vi "Periodic Tasks (Conley Anderson's conflicted copy 2015-02-02).vi"(8 "error in":errorcluster) -> ()   [LabVIEW 2013]
doc: "This VI runs in parallel to other tasks. It can contain as many user-defined periodic loops as you need. These can carry out PID or other sorts of timed response."
uses:
  <vilib>/Rock Robotics/WPI/DriverStation/WPI_DriverStationRobotMode2.ctl
  <vilib>/Rock Robotics/SystemInterfaces/Utilities/FPGA_UtilitiesLED Source.ctl
  <vilib>/Rock Robotics/SystemInterfaces/Utilities/FPGA_UtilitiesLED State.ctl
  <vilib>/Rock Robotics/WPI/Solenoid/WPI_SolenoidValue.ctl
  <vilib>/Rock Robotics/WPI/Relay/WPI_RelayValue.ctl
  <vilib>/Rock Robotics/WPI/Compressor/WPI_CompressorGetSetRefNum.vi
  Robot Global Data.vi
  <vilib>/Rock Robotics/WPI/Joystick/WPI_JoystickGetSetRefNum.vi
  <vilib>/Rock Robotics/WPI/Solenoid/WPI_SolenoidSetEnum.vi
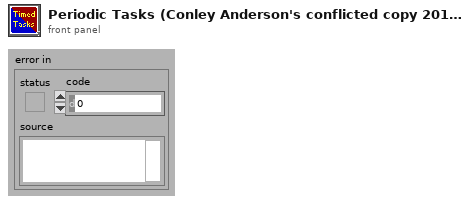
[diagram p1: front panel]
types:
  T1 = typedef "FPGA_UtilitiesLED State.ctl" = enum16{"Off", "On", "Toggle"}
  T2 = typedef "FPGA_UtilitiesLED Source.ctl" = enum16{"User LED", "FPGA LED"}
  T3 = typedef "WPI_AnalogChannelDevRef.ctl" = cluster{"DevStatus":errorcluster, "Analog Module":T4, "Analog Channel":T5}
  T4 = typedef "FPGA_TypedefAnalogModule.ctl" = enum16{"Analog Module 1", "Analog Module 2"}
  T5 = typedef "FPGA_AIChannel.ctl" = enum8{"AI 1", "AI 2", "AI 3", "AI 4", "AI 5", "AI 6", "AI 7", "AI 8", "Invalid"}
  T6 = typedef "WPI_RelayDevRef.ctl" = cluster{"DevStatus":errorcluster, "Relay Channel":T7, "Digital Module":T8, "Relay Direction":T9}
  T7 = typedef "FPGA_DIORelayChannel.ctl" = enum8{"Relay 1", "Relay 2", "Relay 3", "Relay 4", "Relay 5", "Relay 6", "Relay 7", "Relay 8", "Invalid"}
  T8 = typedef "FPGA_TypedefDigitalModule.ctl" = enum16{"Digital Module 1", "Digital Module 2"}
  T9 = typedef "WPI_RelayDirection.ctl" = enum16{"Both directions", "Forward only", "Reverse only"}
  T10 = typedef "WPI_DigitalInputDevRef.ctl" = cluster{"DevStatus":errorcluster, "DIO Channel":T11, "Digital Module":T8}
  T11 = typedef "FPGA_DIOChannel.ctl" = enum8{"DIO 1", "DIO 2", "DIO 3", "DIO 4", "DIO 5", "DIO 6", "DIO 7", "DIO 8", "DIO 9", "DIO 10", "DIO 11", "DIO 12", "DIO 13", "DIO 14", "Invalid"}
  T12 = typedef "WPI_SolenoidDevRef.ctl" = cluster{"DevStatus":errorcluster, "Solenoid Module":T13, "Forward Solenoid Channel":T14, "Reverse Solenoid Channel":T14}
  T13 = typedef "FPGA_TypedefSolenoidModule.ctl" = enum16{"Solenoid Module 1", "Solenoid Module 2"}
  T14 = typedef "WPI_SolenoidChannel.ctl" = enum8{"Solenoid 1", "Solenoid 2", "Solenoid 3", "Solenoid 4", "Solenoid 5", "Solenoid 6", "Solenoid 7", "Solenoid 8", "Invalid"}
  T15 = typedef "WPI_JoystickDevRef.ctl" = cluster{"Device":T16}
  T16 = typedef "WPI_JoystickDeviceEnum.ctl" = enum16{"USB 1", "USB 2", "USB 3", "USB 4", "Kinect 1", "Kinect 2"}
  T17 = typedef "WPI_MotorControlDeviceRef.ctl" = cluster{"DeviceStatus":errorcluster, "Type":enum16{"PWM", "CAN"}, "PWM":cluster{"Digital Module":T8, "PWM Channel":T18, "DeadBand":T19}, "CAN":cluster{"Device Number":u8, "Control Mode":T20, "Semaphore":T21, "Max Vout":dbl}, "Invert":bool, "TransformRef":T22, "InvTransformRef":T22}
  T18 = typedef "FPGA_DIOPWMChannel.ctl" = enum8{"PWM 1", "PWM 2", "PWM 3", "PWM 4", "PWM 5", "PWM 6", "PWM 7", "PWM 8", "PWM 9", "PWM 10", "Invalid"}
  T19 = typedef "WPI_PWMDeadband.ctl" = cluster{"Name":string, "maxPositivePwm":i32, "minPositivePwm":i32, "centerPwm":i32, "maxNegativePwm":i32, "minNegativePwm":i32, "angularRange":u16}
  T20 = typedef "WPI_CANJaguar_ControlMode.ctl" = enum8{"Percent VBus", "Current", "Speed", "Position", "Voltage"}
  T21 = typedef "Semaphore RefNum" = refnum<k1>
  T22 = typedef "WPI_PWMTransform_ConPane.ctl" = refnum<vi>
  T23 = typedef "WPI_CompressorDevRef.ctl" = cluster{"DevStatus":errorcluster, "DigitalInputDevRef":T10, "RelayDevRef":T6}
  T24 = cluster{"JoystickDevRef":T15, "JoystickDevRef":T15, "SolenoidDevRef":T12, "SolenoidDevRef":T12, "RelayDevRef":T6, "RelayDevRef":T6, "RelayDevRef":T6, "MotorControlDevRef":T17, "MotorControlDevRef":T17, "DigitalInputDevRef":T10, "DigitalInputDevRef":T10, "AIDeviceRef":T3, "CompressorDevRef":T23}
  T25 = typedef "WPI_DriverStationRobotMode2.ctl" = enum16{"Autonomous Disabled", "Autonomous Enabled", "Teleop Disabled", "Teleop Enabled", "Timeout", "Finish", "Test Disabled", "Test Enabled"}
  T26 = typedef "WPI_RelayValue.ctl" = enum16{"Off", "On", "Forward", "Reverse"}
  T27 = typedef "WPI_SolenoidValue.ctl" = enum16{"Off", "On", "Forward", "Reverse"}
  T28 = typedef "WPI_JoystickButtonState.ctl" = cluster{"Button 1":bool, "Button 2":bool, "Button 3":bool, "Button 4":bool, "Button 5":bool, "Button 6":bool, "Button 7":bool, "Button 8":bool, "Button 9":bool, "Button 10":bool, "Button 11":bool, "Button 12":bool}
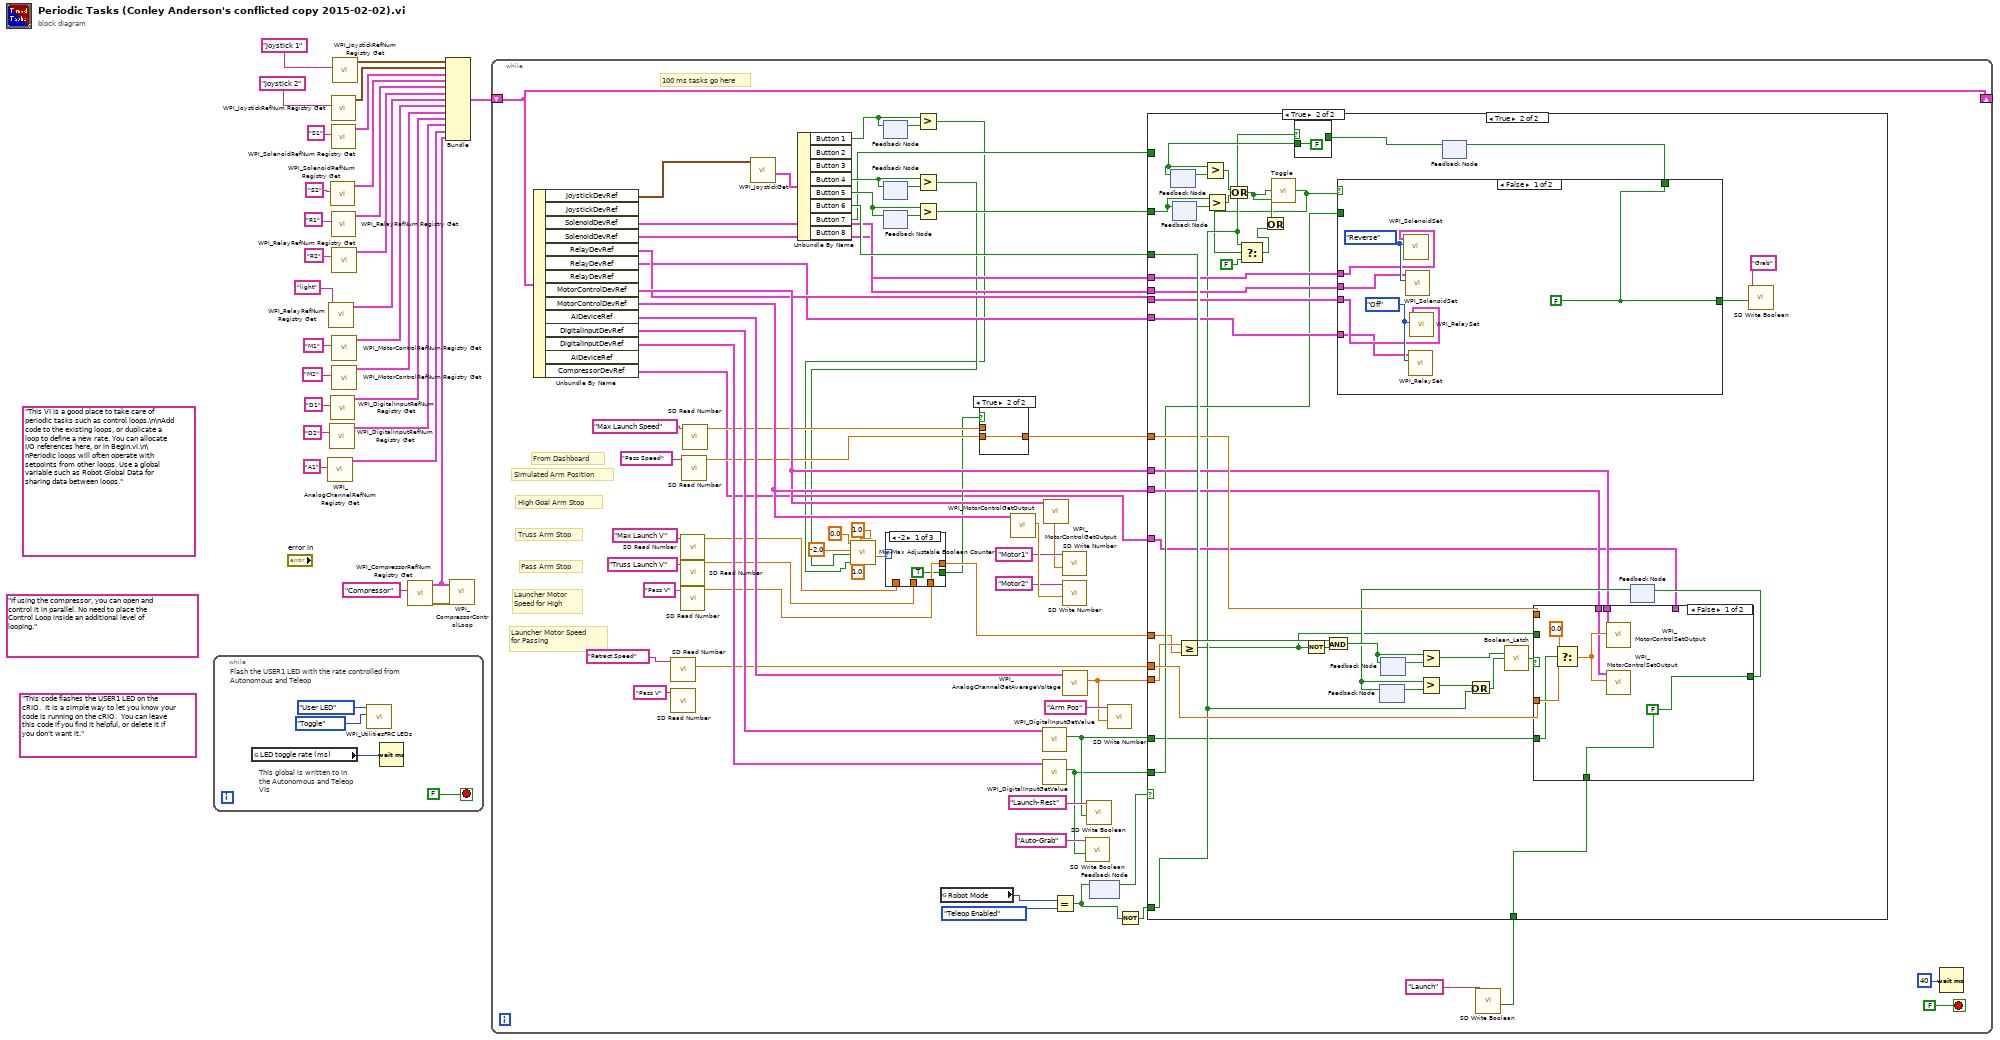
[diagram p0: block diagram]
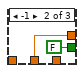
[diagram p3: hidden frame]
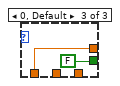
[diagram p4: hidden frame]
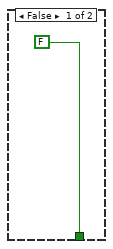
[diagram p5: hidden frame]
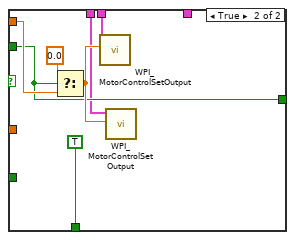
[diagram p7: hidden frame]
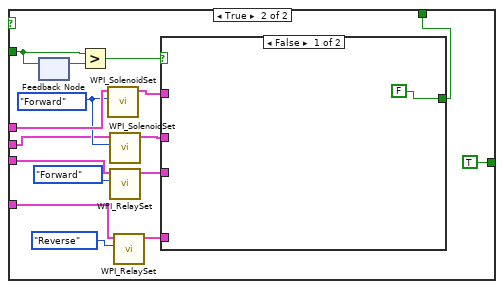
[diagram p8: hidden frame]
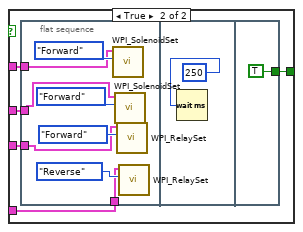
[diagram p9: hidden frame]
diagram:
  (unwired) "If using the compressor, you can open and control it in parallel. No need to place the Control Loop inside an additional level of looping."
  (unwired) "This code flashes the USER1 LED on the cRIO.  It is a simple way to let you know your code is running on the cRIO.  You can leave this code if you find it helpful, or delete it if you don't want it."
  (unwired) "This VI is a good place to take care of periodic tasks such as control loops.\n\nAdd code to the existing loops, or duplicate a loop to define a new rate. You can allocate I/O references here, or in Begin.vi.\n\nPeriodic loops will often operate with setpoints from other loops. Use a global variable such as Robot Global Data for sharing data between loops."
  n1 = while {
    stop <- FALSE stop-if-true
    # "This global is written to in the Autonomous and Teleop VIs"
    # "Flash the USER1 LED with the rate controlled from Autonomous and Teleop"
    n2 = global read "Robot Global Data.vi" "LED toggle rate (ms)"() -> (w29:u32)
    n3 = call <vilib>:"WPI_UtilitiesFRC LEDs.vi"("State"=FPGA_UtilitiesLED_State."Toggle", "LED Type"=FPGA_UtilitiesLED_Source."User LED") -> ()  [unwired: 1 in, 9 out]
    n4 = Wait (ms)(milliseconds to wait=w29) -> ()  [unwired: 1 out]
  }
  n5 = call <vilib>:"WPI_AnalogChannelRefNum Registry Get.vi"("refnum name"="A1") -> ("AIDeviceRef"=w2:T3)  [unwired: 9 in, 1 out]
  n6 = call <vilib>:"WPI_RelayRefNum Registry Get.vi"("refnum name"="light") -> ("RelayDevRef"=w10:T6)  [unwired: 9 in, 1 out]
  n7 = call <vilib>:"WPI_DigitalInputRefNum Registry Get.vi"("refnum name"="D2") -> ("DigitalInputDevRef"=w3:T10)  [unwired: 9 in, 1 out]
  n8 = call <vilib>:"WPI_SolenoidRefNum Registry Get.vi"("refnum name"="S2") -> ("SolenoidDevRef"=w13:T12)  [unwired: 9 in, 1 out]
  n9 = call <vilib>:"WPI_DigitalInputRefNum Registry Get.vi"("refnum name"="D1") -> ("DigitalInputDevRef"=w7:T10)  [unwired: 9 in, 1 out]
  n10 = call <vilib>:"WPI_JoystickRefNum Registry Get.vi"("refnum name"="Joystick 2") -> ("JoystickDevRef"=w5:T15)  [unwired: 1 in, 9 out]
  n11 = call <vilib>:"WPI_SolenoidRefNum Registry Get.vi"("refnum name"="S1") -> ("SolenoidDevRef"=w4:T12)  [unwired: 9 in, 1 out]
  n12 = call <vilib>:"WPI_RelayRefNum Registry Get.vi"("refnum name"="R1") -> ("RelayDevRef"=w12:T6)  [unwired: 9 in, 1 out]
  n13 = call <vilib>:"WPI_RelayRefNum Registry Get.vi"("refnum name"="R2") -> ("RelayDevRef"=w11:T6)  [unwired: 9 in, 1 out]
  n14 = call <vilib>:"WPI_MotorControlRefNum Registry Get.vi"("refnum name"="M1") -> ("MotorControlDevRef"=w9:T17)  [unwired: 9 in, 1 out]
  n15 = call <vilib>:"WPI_MotorControlRefNum Registry Get.vi"("refnum name"="M2") -> ("MotorControlDevRef"=w8:T17)  [unwired: 9 in, 1 out]
  n16 = call <vilib>:"WPI_JoystickRefNum Registry Get.vi"("refnum name"="Joystick 1") -> ("JoystickDevRef"=w6:T15)  [unwired: 1 in, 9 out]
  n17 = call <vilib>:"WPI_CompressorRefNum Registry Get.vi"("refnum name"="Compressor") -> ("error out"=w15:errorcluster, "CompressorDevRef"=w1:T23)  [unwired: 9 in]
  n18 = Bundle("JoystickDevRef"=w6, "JoystickDevRef"=w5, "SolenoidDevRef"=w4, "SolenoidDevRef"=w13, "RelayDevRef"=w12, "RelayDevRef"=w11, "RelayDevRef"=w10, "MotorControlDevRef"=w9, "MotorControlDevRef"=w8, "DigitalInputDevRef"=w7, "DigitalInputDevRef"=w3, "AIDeviceRef"=w2, "CompressorDevRef"=w1) -> (w27:T24)  [unwired: 1 out]
  n19 = call <vilib>:"WPI_CompressorControlLoop.vi"("error in (no error)"=w15, "CompressorDevRef"=w1) -> ()  [unwired: 10 in]
  n20 = while {
    shift-right: [w95] -> _
    shift-left: w27 -> [w95]
    stop <- FALSE stop-if-true
    # "Simulated Arm Position"
    # "Launcher Motor Speed\nfor Passing"
    # "Launcher Motor\nSpeed for High"
    # "Pass Arm Stop"
    # "Truss Arm Stop"
    # "High Goal Arm Stop"
    # "From Dashboard"
    # "100 ms tasks go here"
    n21 = Unbundle By Name(w95) -> ("JoystickDevRef"=w94:T15, "SolenoidDevRef"=w53:T12, "SolenoidDevRef"=w51:T12, "RelayDevRef"=w46:T6, "RelayDevRef"=w45:T6, "MotorControlDevRef"=w75:T17, "MotorControlDevRef"=w76:T17, "AIDeviceRef"=w79:T3, "DigitalInputDevRef"=w81:T10, "DigitalInputDevRef"=w80:T10, "CompressorDevRef"=w41:T23)  [unwired: 3 out]
    n22 = call <vilib>:"SD Read Number.vi"("Name"="Retract Speed") -> ("Numeric"=w47:dbl)  [unwired: 8 in, 2 out]
    n23 = call <vilib>:"SD Read Number.vi"("Name"="Pass V") -> ()  [unwired: 8 in, 3 out]
    n24 = call <vilib>:"SD Read Number.vi"("Name"="Max Launch V") -> ("Numeric"=w63:dbl)  [unwired: 8 in, 2 out]
    n25 = call <vilib>:"SD Read Number.vi"("Name"="Truss Launch V") -> ("Numeric"=w64:dbl)  [unwired: 8 in, 2 out]
    n26 = call <vilib>:"SD Read Number.vi"("Name"="Pass V") -> ("Numeric"=w62:dbl)  [unwired: 8 in, 2 out]
    n27 = call <vilib>:"SD Read Number.vi"("Name"="Pass Speed") -> ("Numeric"=w60:dbl)  [unwired: 8 in, 2 out]
    n28 = call <vilib>:"SD Read Number.vi"("Name"="Max Launch Speed") -> ("Numeric"=w58:dbl)  [unwired: 8 in, 2 out]
    n29 = call <vilib>:"WPI_JoystickGet.vi"("JoystickDevRef"=w94) -> ("Buttons"=w93:T28)  [unwired: 4 in, 2 out]
    n30 = Unbundle By Name(w93) -> ("Button 1"=w91:bool, "Button 4"=w89:bool, "Button 5"=w87:bool, "Button 6"=w70:bool, "Button 7"=w52:bool)  [unwired: 3 out]
    n31 = feedback #1() -> (w92:bool)  [unwired: 1 in]
    n32 = feedback-in #1(w91) -> ()
    n33 = feedback #2() -> (w90:bool)  [unwired: 1 in]
    n34 = feedback-in #2(w89) -> ()
    n35 = feedback #3() -> (w88:bool)  [unwired: 1 in]
    n36 = feedback-in #3(w87) -> ()
    n37 = Greater?(x=w91, y=w92) -> (0:w39:bool)
    n38 = Greater?(x=w89, y=w90) -> (0:w40:bool)
    n39 = call "Min-Max Adjustable Boolean Counter.vi"("Dec Amount"=1.0, "Inc Amount"=1.0, "Decrease"=w39, "Increase"=w40, "Minimum"=-2.0, "Maximum"=0.0) -> ("Counter"=w34:dbl)  [unwired: 5 in]
    n40 = case shown="-2" w34 {
      tunnel: w62 -> [w100 _ _]
      tunnel: w64 -> [_ w102 _]
      tunnel: w63 -> [_ _ w104]
      tunnel: [w100 w102 w104] -> w61
      tunnel: [TRUE FALSE FALSE] -> w49
      frame -2 {
      }
      frame -1 {
      }
      frame 0, Default {
      }
    }
    n41 = Greater?(x=w87, y=w88) -> (0:w86:bool)
    n42 = global read "Robot Global Data.vi" "Robot Mode"() -> (w55:T25)
    n43 = case shown="True" w49 {
      tunnel: w60 -> [_ w98]
      tunnel: [w97 w98] -> w59
      tunnel: w58 -> [w97 _]
      frame False {
      }
      frame True {
      }
    }
    n44 = call <vilib>:"WPI_MotorControlGetOutput.vi"("MotorControlDevRef"=w76) -> ("Output"=w74:dbl)  [unwired: 8 in, 2 out]
    n45 = call <vilib>:"WPI_DigitalInputGetValue.vi"("DigitalInputDevRef"=w81) -> ("Value"=w83:bool)  [unwired: 8 in, 2 out]
    n46 = call <vilib>:"WPI_DigitalInputGetValue.vi"("DigitalInputDevRef"=w80) -> ("Value"=w82:bool)  [unwired: 8 in, 2 out]
    n47 = call <vilib>:"WPI_MotorControlGetOutput.vi"("MotorControlDevRef"=w75) -> ("Output"=w72:dbl)  [unwired: 8 in, 2 out]
    n48 = Equal?(x=w55, y=WPI_DriverStationRobotMode2."Teleop Enabled") -> (x = y?=w42:bool)
    n49 = call <vilib>:"SD Write Number.vi"("Numeric"=w72, "Name"="Motor1") -> ()  [unwired: 8 in, 2 out]
    n50 = call <vilib>:"SD Write Number.vi"("Numeric"=w74, "Name"="Motor2") -> ()  [unwired: 8 in, 2 out]
    n51 = call <vilib>:"WPI_AnalogChannelGetAverageVoltage.vi"("AIDeviceRef"=w79) -> ("Voltage"=w77:dbl)  [unwired: 8 in, 2 out]
    n52 = call <vilib>:"SD Write Boolean.vi"("Boolean"=w82, "Name"="Auto-Grab") -> ()  [unwired: 8 in, 2 out]
    n53 = call <vilib>:"SD Write Boolean.vi"("Boolean"=w83, "Name"="Launch-Rest") -> ()  [unwired: 8 in, 2 out]
    n54 = feedback-in #4(w42) -> ()
    n55 = feedback #4() -> (w44:bool)  [unwired: 1 in]
    n56 = call <vilib>:"SD Write Number.vi"("Numeric"=w77, "Name"="Arm Pos") -> ()  [unwired: 8 in, 2 out]
    n57 = Not(x=w42) -> (.not. x?=w43:bool)
    n58 = case shown="True" w44 {
      tunnel: w86 -> [_ w145]
      tunnel: w83 -> [_ w111]
      tunnel: w82 -> [_ w118]
      tunnel: w77 -> [_ w116]
      tunnel: w76 -> [_ w129]
      tunnel: w75 -> [_ w130]
      tunnel: w70 -> [_ w141]
      tunnel: w61 -> [_ w115]
      tunnel: w59 -> [_ w140]
      tunnel: [FALSE w136] -> w56
      tunnel: w53 -> [_ w128]
      tunnel: w52 -> [_ _]
      tunnel: w51 -> [_ w126]
      tunnel: w47 -> [_ w127]
      tunnel: w46 -> [_ w125]
      tunnel: w45 -> [_ w124]
      tunnel: w43 -> [_ w114]
      tunnel: w41 -> [_ w117]
      frame False {
      }
      frame True {
        n59 = feedback #5() -> (w133:bool)  [unwired: 1 in]
        n60 = feedback #6() -> (w146:bool)  [unwired: 1 in]
        n61 = feedback-in #6(w145) -> ()
        n62 = Greater Or Equal?(x=w116, y=w115) -> (x >= y?=w112:bool)
        n63 = Greater?(x=w145, y=w146) -> (0:w122:bool)
        n64 = Not(x=w112) -> (.not. x?=w142:bool)
        n65 = And(x=w141, y=w142) -> (x .and. y?=w143:bool)
        n66 = feedback #7() -> (w138:bool)  [unwired: 1 in]
        n67 = feedback #8() -> (w144:bool)  [unwired: 1 in]
        n68 = feedback-in #8(w143) -> ()
        n69 = Greater?(x=w143, y=w144) -> (0:w110:bool)
        n70 = feedback #9() -> (w120:bool)  [unwired: 1 in]
        n71 = case shown="True" w114 {
          tunnel: w120 -> [w147 _]
          tunnel: [w147 FALSE] -> w119
          frame False {
          }
          frame True {
          }
        }
        n72 = feedback-in #5(w119) -> ()
        n73 = Greater?(x=w119, y=w133) -> (0:w132:bool)
        n74 = Or(x=w132, y=w122) -> (x .or. y?=w107:bool)
        n75 = call "Toggle.vi"("Input"=w107) -> ("Output"=w106:bool)
        n76 = Select(t=w114, s=w106, f=FALSE) -> (s? t:f=w121:bool)
        n77 = Or(x=w107, y=w121) -> ()  [unwired: 1 out]
        n78 = case shown="False" w106 {
          tunnel: [w168 TRUE] -> w134
          tunnel: [w168 w178] -> w131
          tunnel: w128 -> [w166 w176]
          tunnel: w126 -> [w165 w174]
          tunnel: w125 -> [w164 w173]
          tunnel: w124 -> [w163 w172]
          tunnel: w118 -> [_ w171]
          frame False {
            w169 = WPI_RelayValue."Off" ("RelayValue")
            w168 = FALSE
            w167 = WPI_SolenoidValue."Reverse" ("Value")
            n79 = call-poly <vilib>:"WPI_SolenoidSet.vi"("Value"=w167, "SolenoidDevRef"=w166) -> ()  [unwired: 8 in, 2 out]
            n80 = call-poly <vilib>:"WPI_SolenoidSet.vi"("Value"=w167, "SolenoidDevRef"=w165) -> ()  [unwired: 8 in, 2 out]
            n81 = call <vilib>:"WPI_RelaySet.vi"("RelayValue"=w169, "RelayDevRef"=w163) -> ()  [unwired: 8 in, 2 out]
            n82 = call <vilib>:"WPI_RelaySet.vi"("RelayValue"=w169, "RelayDevRef"=w164) -> ()  [unwired: 8 in, 2 out]
          }
          frame True {
            w175 = WPI_SolenoidValue."Forward" ("Value")
            n83 = feedback #10() -> (w170:bool)  [unwired: 1 in]
            n84 = feedback-in #10(w171) -> ()
            n85 = Greater?(x=w171, y=w170) -> (0:w177:bool)
            n86 = call-poly <vilib>:"WPI_SolenoidSet.vi"("Value"=w175, "SolenoidDevRef"=w176) -> ("SolenoidDevRef"=w182:T12)  [unwired: 8 in, 1 out]
            n87 = call-poly <vilib>:"WPI_SolenoidSet.vi"("Value"=w175, "SolenoidDevRef"=w174) -> ("SolenoidDevRef"=w181:T12)  [unwired: 8 in, 1 out]
            n88 = call <vilib>:"WPI_RelaySet.vi"("RelayValue"=WPI_RelayValue."Forward", "RelayDevRef"=w173) -> ("RelayDevRef"=w180:T6)  [unwired: 8 in, 1 out]
            n89 = call <vilib>:"WPI_RelaySet.vi"("RelayValue"=WPI_RelayValue."Reverse", "RelayDevRef"=w172) -> ("RelayDevRef"=w179:T6)  [unwired: 8 in, 1 out]
            n90 = case shown="False" w177 {
              tunnel: w182 -> [_ w191]
              tunnel: w181 -> [_ w190]
              tunnel: w180 -> [_ w189]
              tunnel: w179 -> [_ w188]
              tunnel: [FALSE w187] -> w178
              frame False {
              }
              frame True {
                n91 = flat-sequence {
                  tunnel: w191 -> [w195]
                  tunnel: w190 -> [w194]
                  tunnel: w189 -> [w193]
                  tunnel: w188 -> [w192]
                  tunnel: [TRUE] -> w187
                  frame #0 {
                    n92 = call-poly <vilib>:"WPI_SolenoidSet.vi"("Value"=WPI_SolenoidValue."Forward", "SolenoidDevRef"=w195) -> ()  [unwired: 8 in, 2 out]
                    n93 = call-poly <vilib>:"WPI_SolenoidSet.vi"("Value"=WPI_SolenoidValue."Forward", "SolenoidDevRef"=w194) -> ()  [unwired: 8 in, 2 out]
                    n94 = call <vilib>:"WPI_RelaySet.vi"("RelayValue"=WPI_RelayValue."Forward", "RelayDevRef"=w193) -> ()  [unwired: 8 in, 2 out]
                    n95 = call <vilib>:"WPI_RelaySet.vi"("RelayValue"=WPI_RelayValue."Reverse", "RelayDevRef"=w192) -> ()  [unwired: 8 in, 2 out]
                  }
                  frame #1 {
                    n96 = Wait (ms)(milliseconds to wait=250) -> ()  [unwired: 1 out]
                  }
                  frame #2 {
                  }
                }
              }
            }
          }
        }
        n97 = feedback-in #9(w131) -> ()
        n98 = feedback #11() -> (w137:bool)  [unwired: 1 in]
        n99 = feedback-in #7(w137) -> ()
        n100 = Greater?(x=w137, y=w138) -> (0:w113:bool)
        n101 = Or(x=w113, y=w114) -> (x .or. y?=w109:bool)
        n102 = call "Boolean_Latch.vi"("Latch Control"=w110, "Reset"=w109) -> ("Latched?"=w108:bool)  [unwired: 13 in]
        n103 = case shown="False" w108 {
          tunnel: w140 -> [_ w161]
          tunnel: w112 -> [_ w159]
          tunnel: [w153 w159] -> w139
          tunnel: [w153 TRUE] -> w136
          tunnel: w130 -> [w151 w157]
          tunnel: w129 -> [w150 w156]
          tunnel: w127 -> [w152 _]
          tunnel: w117 -> [_ _]
          tunnel: w111 -> [w149 _]
          frame False {
            w153 = FALSE
            n104 = Select(t=0.0, s=w149, f=w152) -> (s? t:f=w154:dbl)
            n105 = call <vilib>:"WPI_MotorControlSetOutput.vi"("Output"=w154, "MotorControlDevRef"=w151) -> ()  [unwired: 7 in, 3 out]
            n106 = call <vilib>:"WPI_MotorControlSetOutput.vi"("Output"=w154, "MotorControlDevRef"=w150) -> ()  [unwired: 7 in, 3 out]
          }
          frame True {
            n107 = Select(t=0.0, s=w159, f=w161) -> (s? t:f=w162:dbl)
            n108 = call <vilib>:"WPI_MotorControlSetOutput.vi"("Output"=w162, "MotorControlDevRef"=w157) -> ()  [unwired: 7 in, 3 out]
            n109 = call <vilib>:"WPI_MotorControlSetOutput.vi"("Output"=w162, "MotorControlDevRef"=w156) -> ()  [unwired: 7 in, 3 out]
          }
        }
        n110 = feedback-in #11(w139) -> ()
        n111 = call <vilib>:"SD Write Boolean.vi"("Boolean"=w134, "Name"="Grab") -> ()  [unwired: 8 in, 2 out]
      }
    }
    n112 = call <vilib>:"SD Write Boolean.vi"("Boolean"=w56, "Name"="Launch") -> ()  [unwired: 8 in, 2 out]
    n113 = Wait (ms)(milliseconds to wait=u32 40) -> ()  [unwired: 1 out]
  }
